vi "Tool_Header_Info_Str.vi"(8 "error in (no error)":errorcluster, 10 "Functions":i32, 11 "DefaultDev in":refnum<class "BaseDevice.lvclass">) -> (0 "error out":errorcluster, 1 "HdrInfoStr":string, 2 "InstrumentName":string, 3 "DefaultDev out":refnum<class "BaseDevice.lvclass">)   [LabVIEW 2019, in "BaseDevice.lvclass"]
uses:
  BaseDevice.lvclass
  BaseDevice.lvclass/BaseDevice.ctl
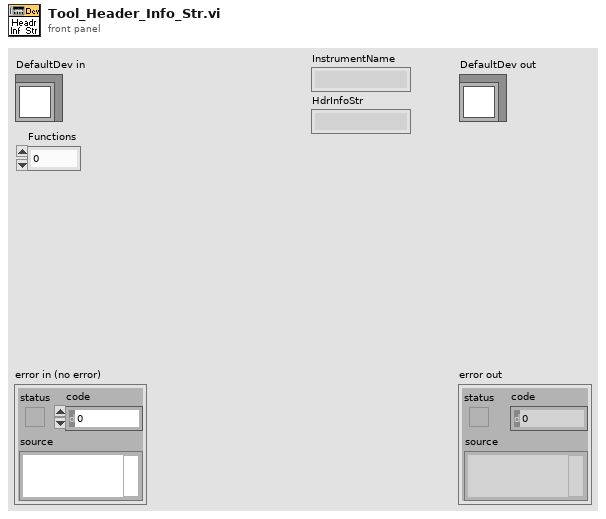
[diagram p1: front panel]
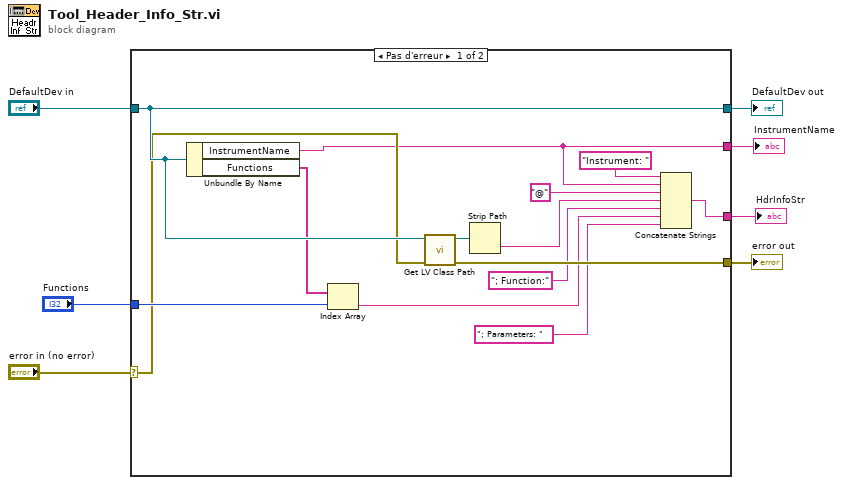
[diagram p0: block diagram]
diagram:
  n1 = case shown="Pas d'erreur" "error in (no error)" {
    selector: "error in (no error)" -> [w10 w23]
    tunnel: [w17 w23] -> w6
    tunnel: [w15 w22] -> w4
    tunnel: "DefaultDev in" -> [w15 w22]
    tunnel: [w9 _] -> w3
    tunnel: [w12 _] -> w2
    tunnel: "Functions" -> [w11 _]
    frame No Error {
      n2 = Unbundle By Name(w15) -> ("InstrumentName"=w9:string, "Functions"=w8:string[])
      n3 = Index Array(array=w8, index=w11) -> (element=w14:string)
      n4 = call <vilib>:"Get LV Class Path.vi"("error in (no error)"=w10, "object"=w15) -> ("error out"=w17:errorcluster, "class path"=w18:path)  [unwired: 8 in]
      n5 = Strip Path(path=w18) -> (name=w20:string)  [unwired: 1 out]
      n6 = Concatenate Strings("Instrument: " ("string"), w9, "@" ("string"), w20, "; Function:" ("Params"), w14, "; Parameters: " ("Params")) -> (w12:string)
    }
    frame Error {
    }
  }
  "error out" <- w6
  "DefaultDev out" <- w4
  "InstrumentName" <- w3
  "HdrInfoStr" <- w2
